vi "mav_main.vi"(8 "error in":errorcluster, 9 "Connection Type":enum32{"TCP", "SERIAL", "UDP"}(ring), 11 "mav_connection_in":T1={"serial"={"baudrate"=115200, "visa in"=""}, "tcp"={"address"="127.0.0.1", "port"=5760}, "udp"={"address"="127.0.0.1", "port"=5760}}) -> (0 "error out":errorcluster)   [LabVIEW 2023]
uses:
  mav_global_var.vi
panel:
  out "stop":bool
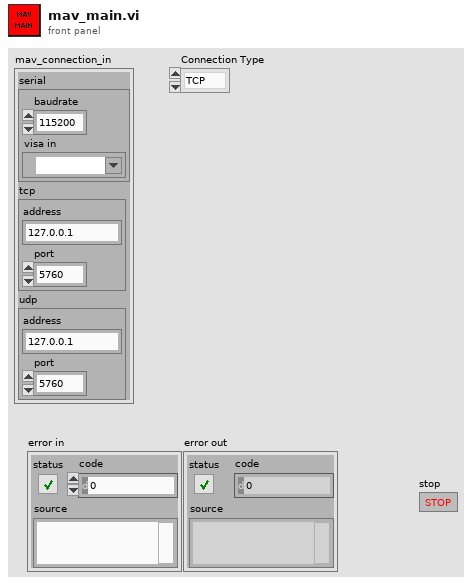
[diagram p1: front panel]
types:
  T1 = cluster{"serial":cluster{"baudrate":u32, "visa in":refnum<visa-resource-name>}, "tcp":cluster{"address":string, "port":u16}, "udp":cluster{"address":string, "port":u16}}
  T2 = cluster{"visa out":refnum<visa-resource-name>, "tcp connection ID":refnum<k5>, "udp connection ID":refnum<k16>}
  T3 = cluster{"len":u8, "incompat_flags":u8, "compat_flags":u8, "seq":u8, "sysid":u8, "compid":u8, "msgid":u32, "magic":u8, "payload":string, "checksum":u16, "signature":string}
  T4 = cluster{"VISA out":refnum<visa-resource-name>, "tcp connection ID":refnum<k5>, "udp connection ID":refnum<k16>}
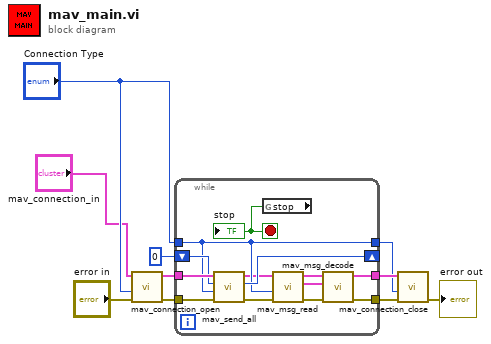
[diagram p0: block diagram]
diagram:
  n1 = call "mav_connection_open.vi"("error in"="error in", "Connection Type"="Connection Type", "mav_connection_in"="mav_connection_in") -> ("error out"=w6:errorcluster, "mav_connection_out"=w7:T2)  [unwired: 7 in]
  n2 = while {
    tunnel: "Connection Type" -> [w14]
    tunnel: [w20] -> w10
    tunnel: [w19] -> w9
    tunnel: [w14] -> w2
    tunnel: w6 -> [w13]
    tunnel: w7 -> [w17]
    shift-right: [w15] -> _
    shift-left: u8 0 ("packet_sequence_in") -> [w16]
    stop <- w18 stop-if-true
    n3 = call "mav_send_all.vi"("error in"=w13, "Connection Type"=w14, "packet_sequence_in"=w16, "mav_connection_in"=w17) -> ("error out"=w12:errorcluster, "packet_sequence_out"=w15:u8, "mav_connection_out"=w11:T2)  [unwired: 5 in]
    n4 = global read "mav_global_var.vi" "stop"() -> (w18:bool)
    "stop" <- w18
    n5 = call "mav_msg_read.vi"("error in"=w12, "Connection Type"=w14, "mav_connection_in"=w11) -> ("error out"=w21:errorcluster, "mav_msg"=w22:T3, "mav_connection_out"=w23:T2)  [unwired: 6 in]
    n6 = call "mav_msg_decode.vi"("mav_connection_in"=w23, "mav_msg"=w22, "error in"=w21) -> ("mav_connection_out"=w20:T4, "error out"=w19:errorcluster)  [unwired: 6 in]
  }
  n7 = call "mav_connection_close.vi"("error in"=w9, "Connection Type"=w2, "mav_connection_in"=w10) -> ("error out"=→"error out":errorcluster)  [unwired: 8 in]
